vi "Create Pattern Script(Addr).vi"(8 "error in (no error)":errorcluster, 10 "Addr":u16, 11 "SPI 3W Pattern Creator in":refnum<class "SPI 3W Pattern Creator.lvclass">) -> (0 "error out":errorcluster, 2 "String":string, 3 "SPI 3W Pattern Creator out":refnum<class "SPI 3W Pattern Creator.lvclass">)   [LabVIEW 2018, in "SPI 3W Pattern Creator.lvlib" / "SPI 3W Pattern Creator.lvclass"]
uses:
  SPI 3W Pattern Creator.lvclass
  Interfaces/Protocol Interface.lvlibp/Interfaces/Protocol Interface/Pin State.ctl
  Interfaces/Protocol Interface.lvlibp/Interfaces/Protocol Interface/Protocol Interface.lvclass
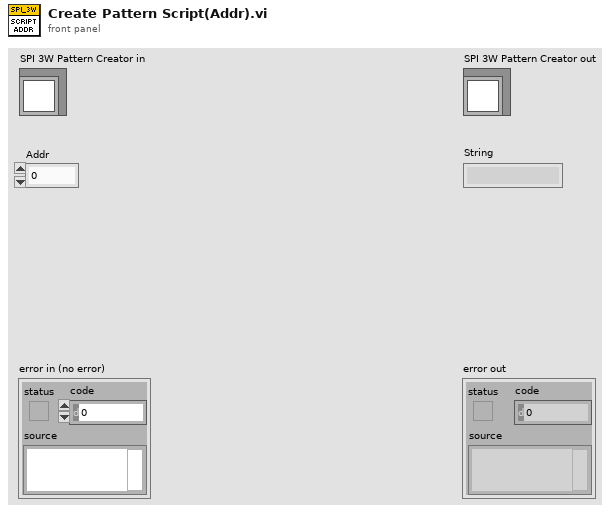
[diagram p1: front panel]
types:
  T1 = typedef "Protocol Interface.lvlibp/Protocol Interface.lvclass/Pin State.ctl" = enum16{"0", "1", "L", "H", "X", "V", "D", "M"}
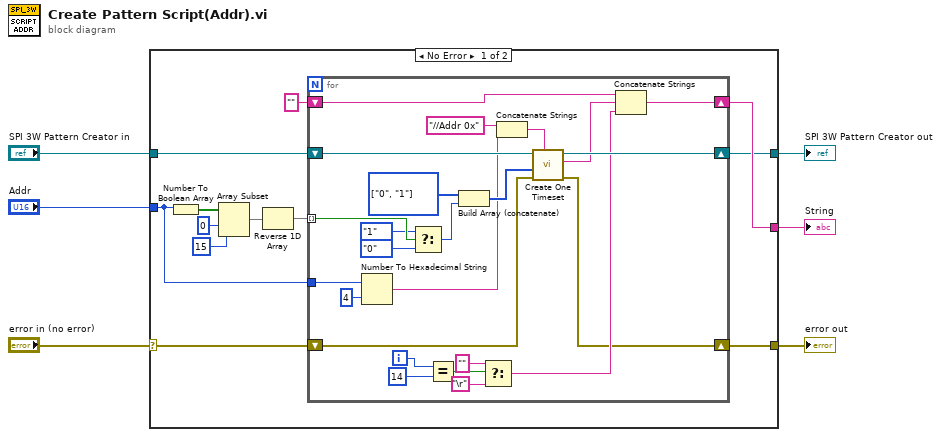
[diagram p0: block diagram]
diagram:
  n1 = case shown="No Error" "error in (no error)" {
    selector: "error in (no error)" -> [w11 w44]
    tunnel: "SPI 3W Pattern Creator in" -> [w12 w43]
    tunnel: "Addr" -> [w13 _]
    tunnel: [w9 _] -> w3
    tunnel: [w8 w43] -> w2
    tunnel: [w7 w44] -> w1
    frame No Error {
      n2 = Number To Boolean Array(number=w13) -> (Boolean array=w18:bool[])
      n3 = Array Subset(array=w18, index=0, length=15) -> (w15:bool[])
      n4 = Reverse 1D Array(array=w15) -> (reversed array=w14:bool[])
      n5 = for {
        tunnel: w14 -> [w40] mode=indexing
        tunnel: w13 -> [w34]
        shift-right: [w29] -> w8
        shift-left: w12 -> [w42]
        shift-right: [w19] -> w7
        shift-left: w11 -> [w41]
        shift-right: [w27] -> w9
        shift-left: "" -> [w26]
        i -> [w25]
        w37 = T1[] [enum."0", enum."1"] items=["0", "1", "L", "H", "X", "V", "D", "M"] ("PinStates")
        n6 = Number To Hexadecimal String(1:i16 4 ("width (-)"), 2:w34) -> (0:w30:string)
        n7 = Select(t=Pin_State."1" ("PinState"), s=w40, f=Pin_State."0") -> (s? t:f=w36:T1)
        n8 = Equal?(x=w25, y=14) -> (x = y?=w23:bool)
        n9 = Build Array (concatenate)(w37, w36) -> (w35:T1[])
        n10 = Select(t="", s=w23, f="\r") -> (s? t:f=w20:string)
        n11 = Concatenate Strings("//Addr 0x" ("string"), w30) -> (w32:string)
        n12 = call-dynamic "Create One Timeset.vi"("Notes"=w32, "error in (no error)"=w41, "PinStates"=w35, "SPI 3W Pattern Creator in"=w42) -> ("error out"=w19:errorcluster, "String  out"=w28:string, "SPI 3W Pattern Creator out"=w29:refnum<class "SPI 3W Pattern Creator.lvclass">)  [unwired: 5 in]
        n13 = Concatenate Strings(w26, w28, w20) -> (w27:string)
      }
    }
    frame Error {
    }
  }
  "error out" <- w1
  "SPI 3W Pattern Creator out" <- w2
  "String" <- w3
